vi "Find Visible Trees.vi"(0 "Tree Grid":i32[][](array[numeric]), 1 "Use":enum16{"Set", "Array"}(ring)) -> (2 "Visible Trees (set)":set{cdb}(c389), 3 "Visible Trees (array)":cdb[](array[numeric]))   [LabVIEW 2020, in "AoC 2022.lvlib"]
uses:
  AoC 2022.lvlib
  ad10f804-0bce-4074-b32b-afe5c27571ce.vi
panel:
  out "Debug: Traverse Orders":T1(array[cluster])
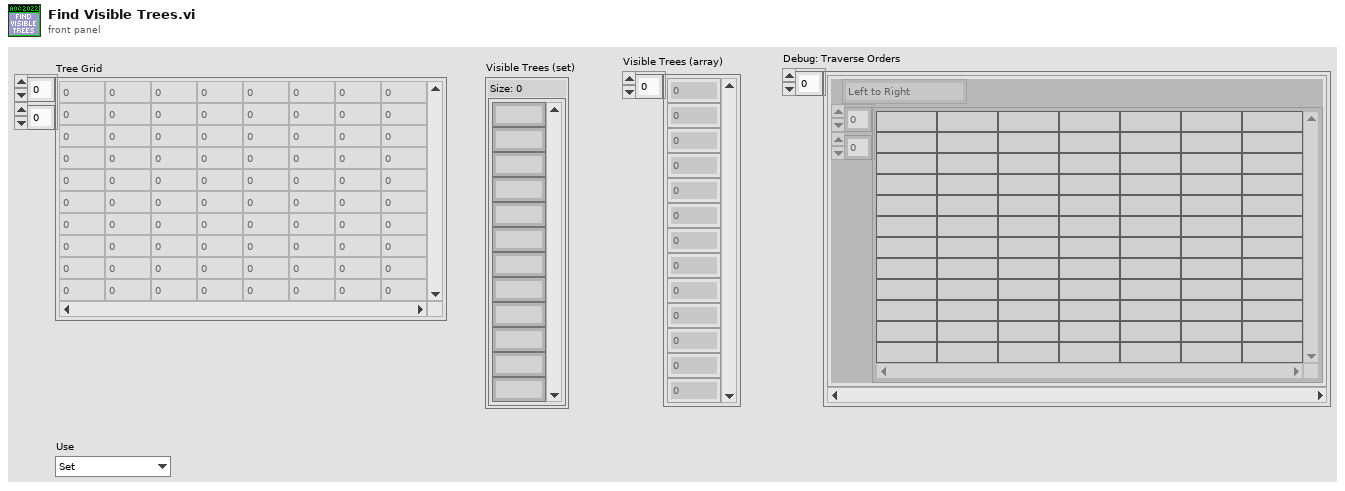
[diagram p1: front panel]
types:
  T1 = cluster{"enum":enum16{"Left to Right", "Right to Left", "Top to Bottom", "Bottom to Top"}, string[][]}[]
  T2 = enum16{"Left to Right", "Right to Left", "Top to Bottom", "Bottom to Top"}
  T3 = enum16{"Left to Right", "Right to Left", "Top to Bottom", "Bottom to Top"}[]
  T4 = cluster{"enum":enum16{"Left to Right", "Right to Left", "Top to Bottom", "Bottom to Top"}, string[][]}
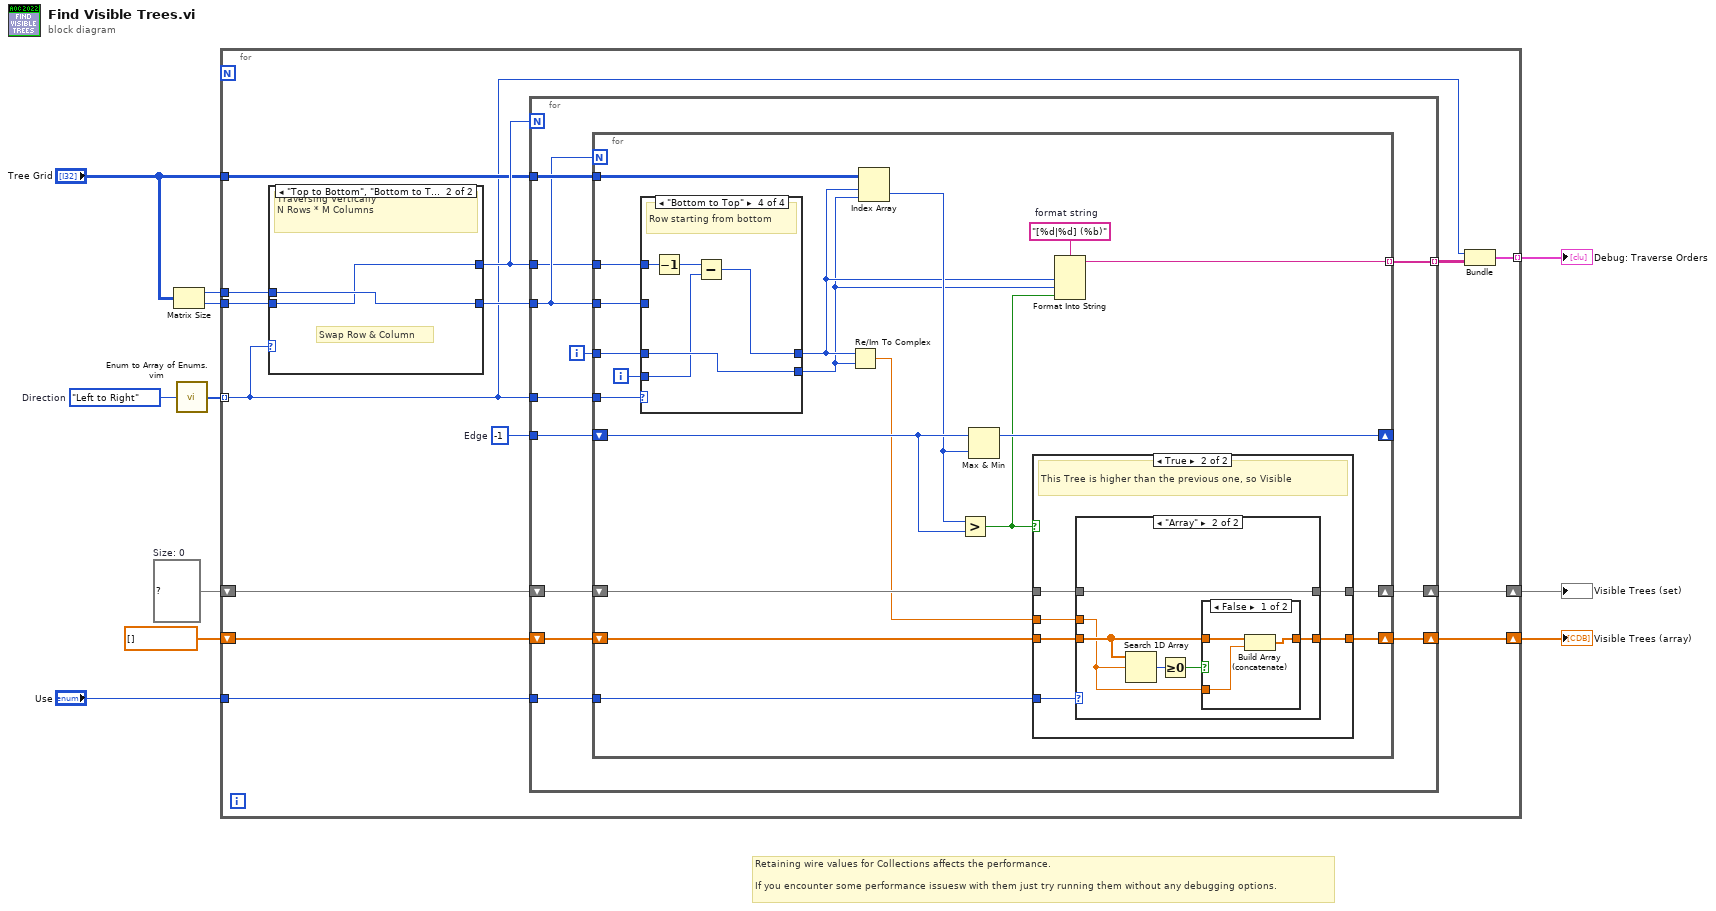
[diagram p0: block diagram]
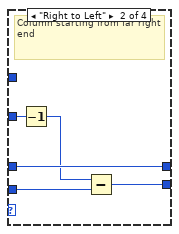
[diagram p3: hidden frame]
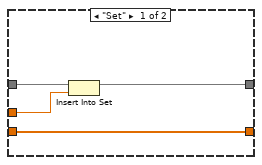
[diagram p6: hidden frame]
diagram:
  w10 = T2."Left to Right"  # Direction
  w9 = set{cdb} {}  # Size: 0
  # "Retaining wire values for Collections affects the performance.\n\nIf you encounter some performance issuesw with them just try running them without any debugging options."
  n1 = Matrix Size(0:"Tree Grid") -> (1:w6:i32, 2:w7:i32)
  n2 = call "Enum to Array of Enums.vim"("enum"=w10) -> ("array of enums"=w5:T3)
  n3 = for {
    tunnel: w5 -> [w17] mode=indexing
    tunnel: "Tree Grid" -> [w21]
    tunnel: w7 -> [w19]
    tunnel: w6 -> [w18]
    shift-right: [w25] -> w11
    shift-left: w9 -> [w23]
    tunnel: [w15] -> w4 mode=indexing
    shift-right: [w13] -> w2
    shift-left: cdb[] [] -> [w14]
    tunnel: "Use" -> [w12]
    w22 = -1  # Edge
    n4 = case shown="\"Top to Bottom\", \"Bottom to Top\"" w17 {
      tunnel: w18 -> [w94 w97]
      tunnel: w19 -> [w95 w96]
      tunnel: [w95 w97] -> w20
      tunnel: [w94 w96] -> w24
      frame "Left to Right", "Right to Left" {
        # "Traversing Horizontaly\nM Rows * N Columns"
      }
      frame "Top to Bottom", "Bottom to Top" {
        # "Swap Row & Column"
        # "Traversing Vertically\nN Rows * M Columns"
      }
    }
    n5 = for {
      N: w24 -> [_]
      tunnel: w20 -> [w31]
      tunnel: w21 -> [w37]
      tunnel: w17 -> [w35]
      tunnel: w22 -> [w34]
      shift-right: [w32] -> w25
      shift-left: w23 -> [w33]
      tunnel: w24 -> [w30]
      tunnel: [w29] -> w16 mode=indexing
      shift-right: [w27] -> w13
      shift-left: w14 -> [w28]
      tunnel: w12 -> [w26]
      i -> [w36]
      n6 = for {
        N: w31 -> [_]
        tunnel: w37 -> [w57]
        tunnel: w36 -> [w55]
        tunnel: w35 -> [w56]
        shift-right: [w51] -> _
        shift-left: w34 -> [w53]
        shift-right: [w49] -> w32
        shift-left: w33 -> [w50]
        tunnel: w31 -> [w47]
        tunnel: w30 -> [w46]
        tunnel: [w43] -> w29 mode=indexing
        shift-right: [w39] -> w27
        shift-left: w28 -> [w40]
        tunnel: w26 -> [w38]
        i -> [w54]
        w44 = "[%d|%d] (%b)"  # format string
        n7 = case shown="\"Bottom to Top\"" w56 {
          tunnel: [w58 w64 w66 w67] -> w45
          tunnel: w55 -> [w58 w64 w65 w71]
          tunnel: [w59 w60 w65 w71] -> w41
          tunnel: w54 -> [w59 w62 w66 w68]
          tunnel: w47 -> [_ w63 _ _]
          tunnel: w46 -> [_ _ _ w70]
          frame "Left to Right" {
            # "Normal Flow"
          }
          frame "Right to Left" {
            # "Column starting from far right end"
            n8 = Decrement(x=w63) -> (x-1=w61:i32)
            n9 = Subtract(x=w61, y=w62) -> (x-y=w60:i32)
          }
          frame "Top to Bottom" {
            # "Normal Flow"
          }
          frame "Bottom to Top" {
            # "Row starting from bottom"
            n10 = Decrement(x=w70) -> (x-1=w69:i32)
            n11 = Subtract(x=w69, y=w68) -> (x-y=w67:i32)
          }
        }
        n12 = Re/Im To Complex(1:w41, 2:w45) -> (0:w48:cdb)
        n13 = Index Array(array=w57, index (row)=w45, index (col)=w41) -> (element=w52:i32)
        n14 = Greater?(x=w52, y=w53) -> (0:w42:bool)
        n15 = Max & Min(x=w53, y=w52) -> (max(x,y)=w51:i32)  [unwired: 1 out]
        n16 = case shown="True" w42 {
          tunnel: w48 -> [_ w79]
          tunnel: [w73 w78] -> w49
          tunnel: w50 -> [w73 w77]
          tunnel: w40 -> [w72 w76]
          tunnel: [w72 w75] -> w39
          tunnel: w38 -> [_ w74]
          frame False {
          }
          frame True {
            # "This Tree is higher than the previous one, so Visible"
            n17 = case shown="\"Array\"" w74 {
              tunnel: w79 -> [w83 w85]
              tunnel: [w82 w89] -> w78
              tunnel: w77 -> [w81 w89]
              tunnel: w76 -> [w80 w86]
              tunnel: [w80 w84] -> w75
              frame "Set" {
                n18 = Insert Into Set(10:w83, 11:w81) -> (3:w82:set{cdb})  [unwired: 1 out]
              }
              frame "Array" {
                n19 = Search 1D Array(1D array=w86, element=w85) -> (index of element=w88:i32)  [unwired: 1 in]
                n20 = Greater Or Equal To 0?(x=w88) -> (x >= 0?=w87:bool)
                n21 = case shown="False" w87 {
                  tunnel: w86 -> [w92 w93]
                  tunnel: w85 -> [w91 _]
                  tunnel: [w90 w93] -> w84
                  frame False {
                    n22 = Build Array (concatenate)(w92, w91) -> (w90:cdb[])
                  }
                  frame True {
                  }
                }
              }
            }
          }
        }
        n23 = Format Into String(format string=w44, w45, w41, w42) -> (resulting string=w43:string)  [unwired: 2 in, 1 out]
      }
    }
    n24 = Bundle("enum"=w17, w16) -> (w15:T4)  [unwired: 1 in]
  }
  "Visible Trees (set)" <- w11
  "Debug: Traverse Orders" <- w4
  "Visible Trees (array)" <- w2
